vi "New Configuration File Binding.vi"(9 "Key Name":string, 10 "Section Name":string, 11 "Config File Refnum":T1) -> (0 "error out":errorcluster, 3 "ConfigurationFileBinding":refnum<class "ConfigurationFileBinding.lvclass">)   [LabVIEW 2015, in "Transport.lvlib" / "ConfigurationFileBinding.lvclass"]
doc: "<License>\nCopyright © 2017 Composed Systems, LLC | All rights reserved\nwww.composed.io\n\nAuthor: Ethan Stern <ethan.stern@composed.io>\n\nThis software is provided \"AS IS\" WITHOUT WARRANTIES, either express or implied, AND IS FOR EDUCATIONAL PURPOSES ONLY.\n</License>"
uses:
  ConfigurationFileBinding.lvclass
  <vilib>/Utility/config.llb/Config Data RefNum.ctl
  ConfigurationFileBinding.lvclass/ConfigurationFileBinding.ctl
  <vilib>/Utility/config.llb/NI_LVConfig.lvlib
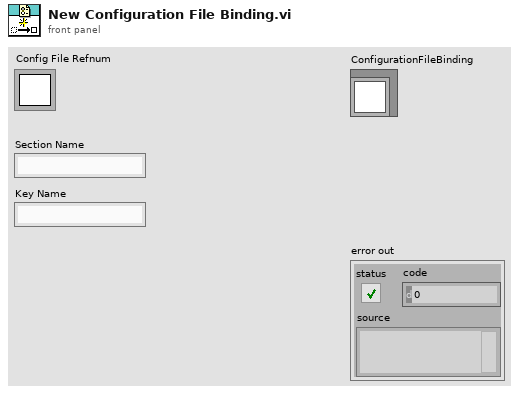
[diagram p1: front panel]
types:
  T1 = typedef "NI_LVConfig.lvlib/Config Data RefNum.ctl" = refnum<k1>
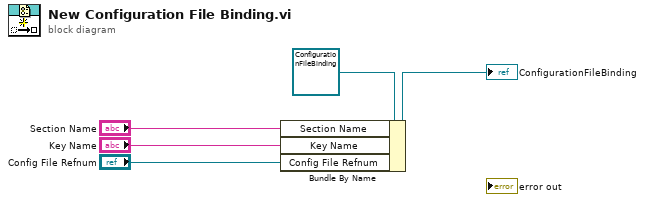
[diagram p0: block diagram]
diagram:
  n1 = Bundle By Name(cluster=refnum<class "ConfigurationFileBinding.lvclass"> refnum ("TerminalReference in"), "Section Name"="Section Name", "Key Name"="Key Name", "Config File Refnum"="Config File Refnum") -> (→"ConfigurationFileBinding":refnum<class "ConfigurationFileBinding.lvclass">)
